vi "FindWorkingZDistance2.vi"(8 "error in":errorcluster, 11 "Images Directory":path=path "C:/Users/Aerotech/Documents/Stave Assembly Records/2017-03-06/autofocusing") -> (0 "error out":errorcluster, 2 "Uncertainty on optimized Z":dbl, 3 "Optimized Z":dbl)   [LabVIEW 2016]
uses:
  <vilib>/Utility/file.llb/Read Delimited Spreadsheet (DBL).vi
  <vilib>/regexp/Match Regular Expression.xnode
  <vilib>/vision/NI_Vision_Development_Module.lvlib
panel:
  in  "Tab Control: Plots":T1(tab)
  out "Waveform Graph":T2(graph)
  out "Histogram Report":T3 {"Standard  Variation" format="%.2f"; "Mean Value" format="%.2f"; "Interval Width" format="%.2f"; "Starting Value" format="%.2f"; "Maximal Value" format="%.2f"; "Minimal Value" format="%.2f"}
  out "SD(I) vs Z":T4(graph)
  out "Location of minimum":dbl
  out "Uncertainty on minimum location":dbl
  in  "Tab Control":enum32{"Images", "Results & error handling"}(tab)=enum."Results & error handling"
  out "Capture coordinates":dbl[][](array[numeric])
  out "Search running?":bool
  out "Finished!":bool
  out "Processing Image #":i32
  out "Search image out":T5(plugin-control)
  in  "Naming Convention":string="*.png"
  in  "Minimization inputs":T6={"Minimizing alg"=0, "Search start"=0.0, "Search end"=1.0, "Search accuracy"=1e-08, "Step type"=0} {"Step type" items=["fixed function", "modified function"]; "Search accuracy" format="%.2e"; "Search end" format="%.2f"; "Search start" format="%.2f"; "Minimizing alg" items=["Golden Section Search", "Brent with Derivatives"]}
  # "FIND CAMERA WORKING DISTANCE Brandeis University - Brookhaven National Laboratory * ATLAS Phase II Inner Tracker Upgrade"
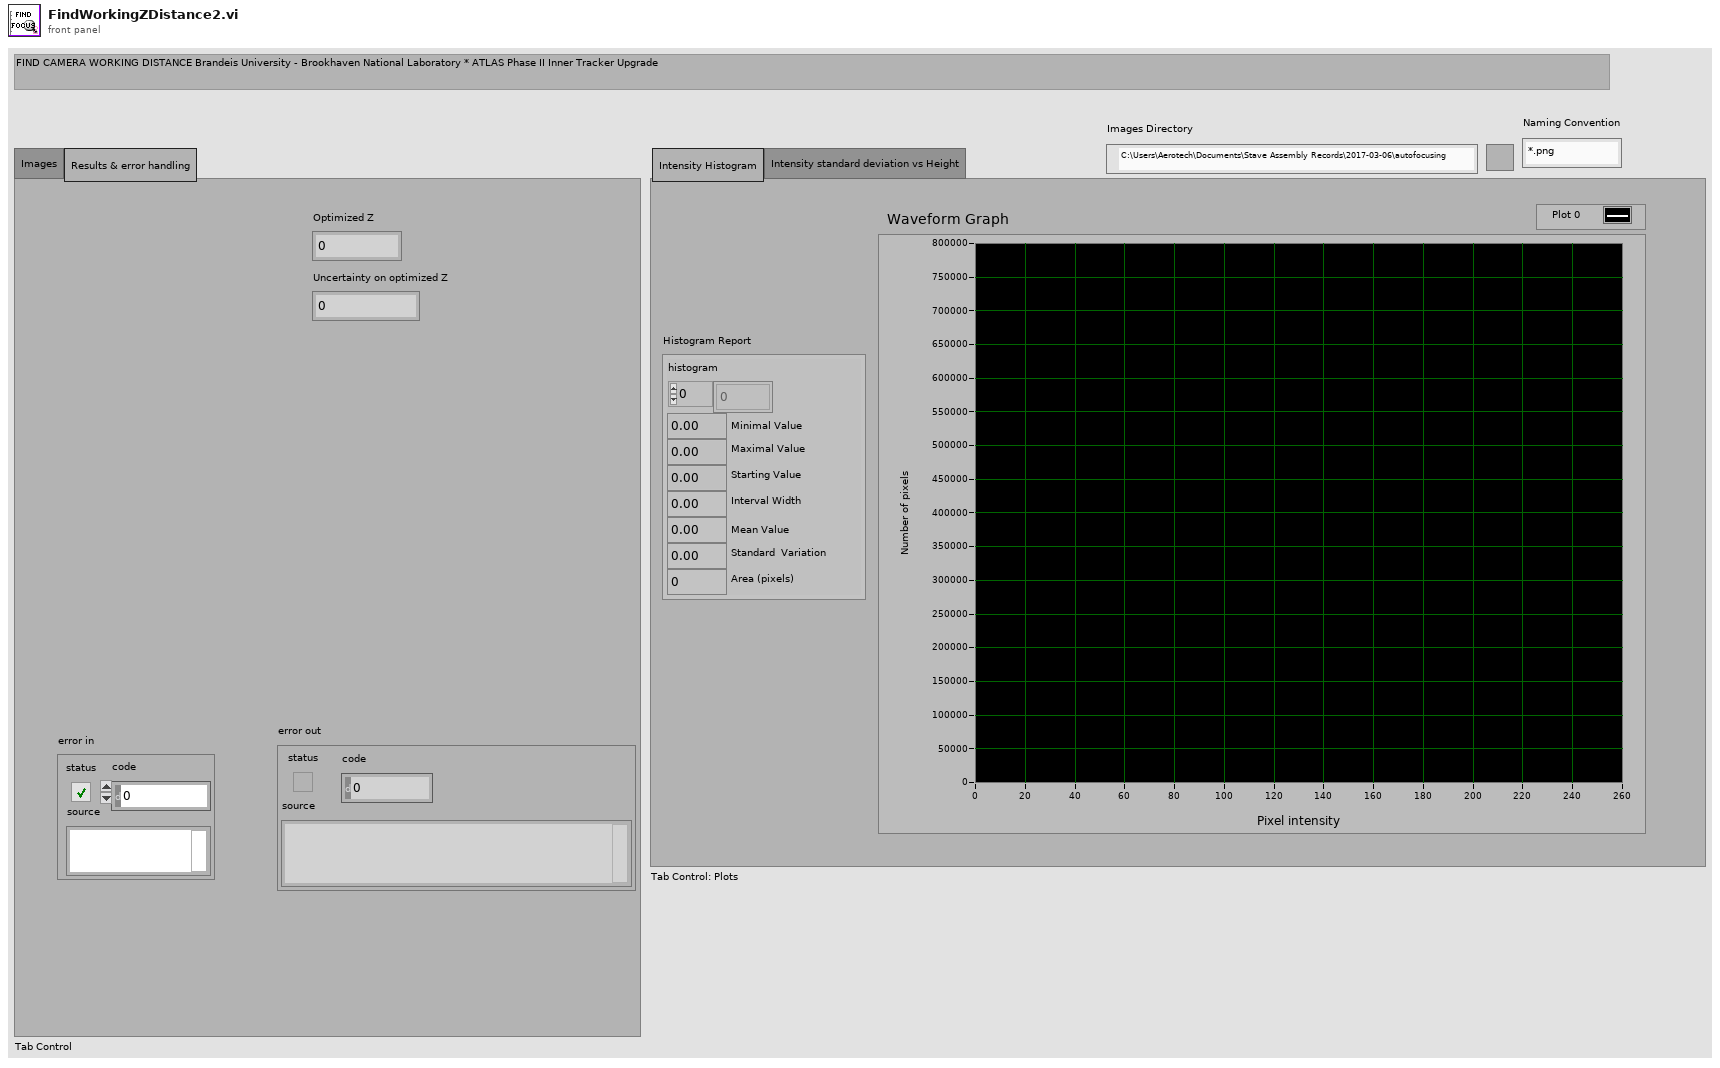
[diagram p1: front panel]
types:
  T1 = enum32{"Intensity Histogram", "Intensity standard deviation vs Height"}
  T2 = cluster{"Starting Value":sgl, "Incremental Value":sgl, "Histogram":u32[]}
  T3 = cluster{"histogram":u32[], "Minimal Value":sgl, "Maximal Value":sgl, "Starting Value":sgl, "Interval Width":sgl, "Mean Value":sgl, "Standard  Variation":sgl, "Area (pixels)":i32}
  T4 = cluster{"Radius bins":dbl[], "Best Gaussian Fit":dbl[]}[]
  T5 = typedef "IMAQ Image.ctl" = refnum<image>
  T6 = cluster{"Minimizing alg":u16, "Search start":dbl, "Search end":dbl, "Search accuracy":dbl, "Step type":u16}
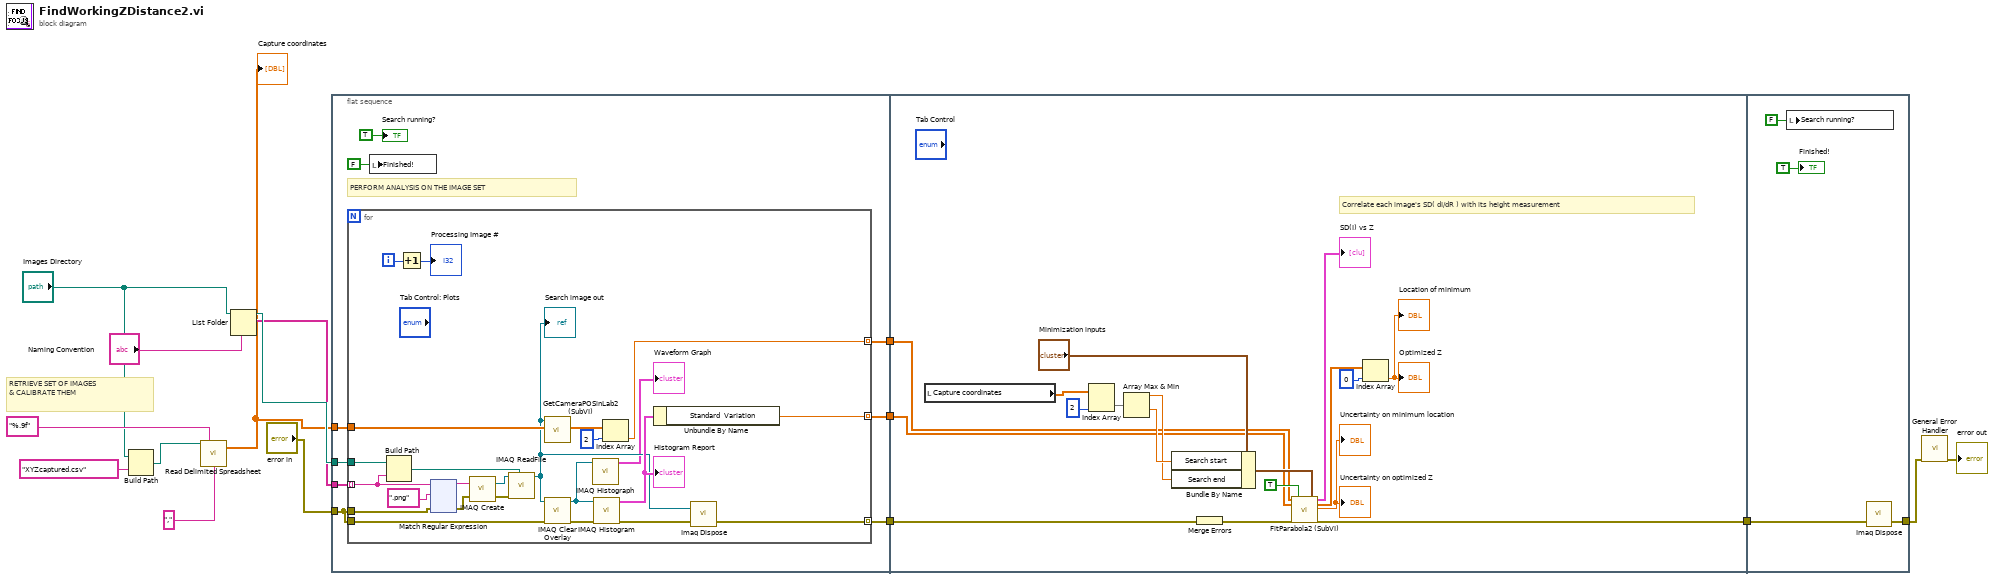
[diagram p0: block diagram]
diagram:
  # "RETRIEVE SET OF IMAGES\n& CALIBRATE THEM"
  n1 = Build Path(base path="Images Directory", name or relative path="XYZcaptured.csv") -> (appended path=w11:path)
  n2 = call-poly <vilib>:"Read Delimited Spreadsheet.vi"("file path (dialog if empty)"=w11, "format (%.3f)"="%.9f", "delimiter (\\t)"="," ("delimiter (\\t)")) -> ("all rows"=w3:dbl[][])  [unwired: 7 in, 5 out]
  "Capture coordinates" <- w3
  n3 = List Folder(path="Images Directory", pattern="Naming Convention") -> (path out=w5:path, filenames=w4:string[])  [unwired: 2 in, 2 out]
  n4 = flat-sequence {
    tunnel: "error in" -> [w19]
    tunnel: w3 -> [w23]
    tunnel: [w22] -> w14
    tunnel: [w21] -> w12
    tunnel: w4 -> [w20]
    tunnel: w5 -> [w18]
    tunnel: [w17] -> w1
    tunnel: [w176] -> w15
    tunnel: w14 -> [w181]
    tunnel: w12 -> [w168]
    tunnel: w1 -> [w164]
    tunnel: [w182] -> w2
    tunnel: w15 -> [w183]
    frame #0 {
      # "PERFORM ANALYSIS ON THE IMAGE SET"
      n5 = for {
        tunnel: w19 -> [w47]
        tunnel: w23 -> [w48]
        tunnel: [w46] -> w22 mode=indexing
        tunnel: [w30] -> w17 mode=indexing
        tunnel: [w45] -> w21 mode=indexing
        tunnel: w20 -> [w37] mode=indexing
        tunnel: w19 -> [w36]
        tunnel: w18 -> [w35]
        i -> [w34]
        n6 = Build Path(base path=w35, name or relative path=w37) -> (appended path=w41:path)
        n7 = Increment(x=w34) -> (x+1=→"Processing Image #":i32)
        n8 = xnode "Match Regular Expression"("input string"=w37, "regular expression"=".png", "error in"=w36) -> ("before match"=w39:string, "error out"=w38:errorcluster)  [unwired: 3 in, 3 out]
        n9 = call "IMAQ Create"("Image Name"=w39, "error in (no error)"=w38) -> ("New Image"=w42:T5, "error out"=w43:errorcluster)  [unwired: 3 in]
        n10 = call "IMAQ ReadFile"("File Path"=w41, "error in (no error)"=w43, "Image"=w42) -> ("Image Out"=w29:T5)  [unwired: 4 in, 4 out]
        "Search image out" <- w29
        n11 = call "GetCameraPOSinLab2 (SubVI).vi"("Loaded array"=w48, "Refnum in"=w29) -> ("Image coordinates in lab frame"=w49:dbl[])  [unwired: 7 in, 2 out]
        n12 = call "IMAQ Clear Overlay"("error in (no error)"=w47, "Image"=w29) -> ("error out"=w32:errorcluster, "Image Out"=w27:T5)  [unwired: 8 in]
        n13 = call "IMAQ Histograph"("Image"=w27) -> ("Histogram Graph"=→"Waveform Graph":T2)  [unwired: 7 in, 3 out]
        n14 = call "IMAQ Histogram"("error in (no error)"=w32, "Image"=w27) -> ("error out"=w28:errorcluster, "Histogram Report"=w31:T3)  [unwired: 8 in]
        "Histogram Report" <- w31
        n15 = Index Array(array=w49, index=2 ("disabled index (col)")) -> (element=w45:dbl)
        n16 = Unbundle By Name(w31) -> ("Standard  Variation"=w30:sgl)
        n17 = call "Imaq Dispose"("Image"=w29, "error in (no error)"=w28) -> ("error out"=w46:errorcluster)  [unwired: 4 in]
      }
      n18 = local write "Finished!"(FALSE ("Review")) -> ()
      "Search running?" <- TRUE ("Search running?")
    }
    frame #1 {
      # "Correlate each image's SD( dI/dR ) with its height measurement"
      n19 = local read "Capture coordinates"() -> (w175:dbl[][])
      n20 = Index Array(array=w175, index (col)=2 ("disabled index (col)")) -> (element=w173:dbl[])  [unwired: 1 in]
      n21 = Array Max & Min(array=w173) -> (max value=w171:dbl, min value=w172:dbl)  [unwired: 2 out]
      n22 = Bundle By Name(cluster="Minimization inputs", "Search start"=w172, "Search end"=w171) -> (w169:T6)
      n23 = Merge Errors(w181) -> (w177:errorcluster)
      n24 = call "FitParabola2 (SubVI).vi"("x values"=w168, "y values"=w164, "error in"=w177, "Use all points"=TRUE, "Minimization inputs"=w169) -> ("Plot with quadratic fit"=→"SD(I) vs Z":T4, "Minima"=w179:dbl[], "Uncertainty on minimum"=→"Uncertainty on optimized Z" →"Uncertainty on minimum location":dbl, "error out"=w176:errorcluster)  [unwired: 11 in]
      n25 = Index Array(array=w179, index=0) -> (element=→"Optimized Z" →"Location of minimum":dbl)
    }
    frame #2 {
      n26 = local write "Search running?"(FALSE ("Search running?")) -> ()
      n27 = call "Imaq Dispose"("error in (no error)"=w183) -> ("error out"=w182:errorcluster)  [unwired: 5 in]
      "Finished!" <- TRUE ("Review")
    }
  }
  n28 = call <vilib>:"General Error Handler.vi"("error in (no error)"=w2) -> ("error out"=→"error out":errorcluster)  [unwired: 10 in, 4 out]
